vi "Pfeiffer Vacuum Digiline Read Data.vi"(8 "error in (no error)":errorcluster, 9 "DigiLine-Cluster":T1={"Parameter"=0, "Parameter\nread only<->describe"=FALSE, "Correction facktor\n(0,20 - 9,90) "=1.0, "Pressure set point (mbar)\n0 ==> ur (p<1,0e-4 mbar)\n1 - 2050 mbar"=0} {"Pressure set point (mbar)\n0 ==> ur (p<1,0e-4 mbar)\n1 - 2050 mbar" min=0 max=2050 step=1; "Correction facktor\n(0,20 - 9,90)" min=0.2 max=9.9 step=0.01 format="%.2f"; "Parameter" items=[" Pressure  [mbar]", " Correction factor 1", " Correction factor 2 (Bayard Albert)", " Actual error code (read only)", " Software version Transmitter  (read only)", " Unit type Transmitter (read only)"]}, 10 "Adress of unit":u16=1 min=1 max=999 step=1, 11 "VISA session in":refnum<visa-resource-name>) -> (0 "error out":errorcluster, 3 "response (data)":string)   [LabVIEW 2016]
doc: "This VI is an example of how to use the Pfeiffer Vacuum subVIs programmatically. This VI first initializes the instrument, takes measurements, then closes the instrument."
uses:
  Public/DigiLine/Digiline - Cluster.ctl
  Pfeiffer Vacuum.lvlib
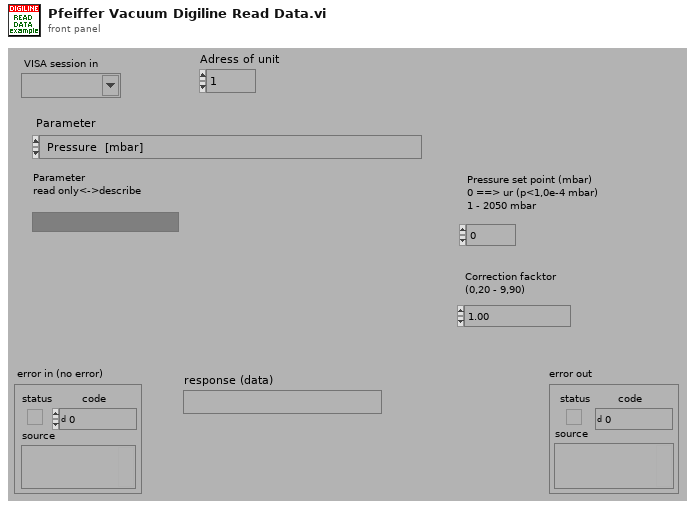
[diagram p1: front panel]
types:
  T1 = typedef "Pfeiffer Vacuum.lvlib/Digiline - Cluster.ctl" = cluster{"Parameter":u16, "Parameter\nread only<->describe":bool, "Correction facktor\n(0,20 - 9,90) ":sgl, "Pressure set point (mbar)\n0 ==> ur (p<1,0e-4 mbar)\n1 - 2050 mbar":i16}
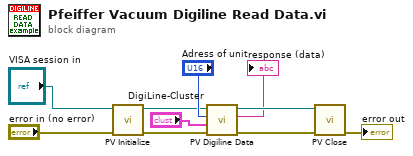
[diagram p0: block diagram]
diagram:
  n1 = call "PV Initialize.vi"("error in (no error)"="error in (no error)", "VISA session in"="VISA session in") -> ("error out"=w4:errorcluster, "VISA session out"=w3:refnum<visa-resource-name>)  [unwired: 8 in]
  n2 = call "PV Digiline Data.vi"("error in (no error)"=w4, "DigiLine-Cluster"="DigiLine-Cluster", "Adress of unit"="Adress of unit", "VISA session"=w3) -> ("error out"=w10:errorcluster, "response (data)"=→"response (data)":string, "dup VISA session"=w9:refnum<visa-resource-name>)  [unwired: 5 in]
  n3 = call "PV Close.vi"("VISA session"=w9, "error in (no error)"=w10) -> ("error out"=→"error out":errorcluster)  [unwired: 13 in]
